vi "TimingLoop.vi"(8 "Error In":errorcluster, 11 "Message Queues":T1) -> (0 "Error Out":errorcluster)   [LabVIEW 2017, in "Server.lvlib" / "Timing.lvlib"]
doc: "This Loop is responsible for sending cyclic messages to MHL."
uses:
  Timing.lvlib
  Message Queue/CommReferences.ctl
  Message Queue/MessageCluster.ctl
  MessageSetList.ctl
  MessageSet.ctl
  <vilib>/Utility/error.llb/Error Cluster From Error Code.vi
  Message Queue/EnqueueMessage(Single).vi
  <vilib>/ErrorRing/Error Ring.xnode
  Message Queue/Message Queue.lvlib
  ErrorLogger/ErrorLogger.lvlib
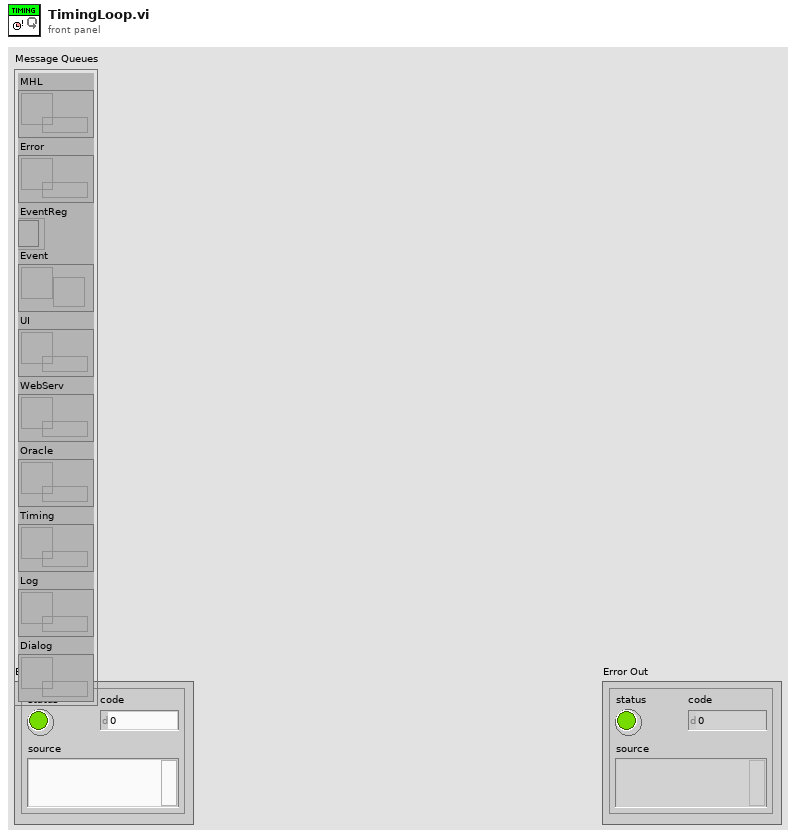
[diagram p1: front panel]
types:
  T1 = typedef "Server.lvlib/Message Queue.lvlib/CommReferences.ctl" = cluster{"MHL":refnum<queue>, "Error":refnum<queue>, "EventReg":refnum<event-registration>, "Event":refnum<user-event>, "UI":refnum<queue>, "WebServ":refnum<queue>, "Oracle":refnum<queue>, "Timing":refnum<queue>, "Log":refnum<queue>, "Dialog":refnum<queue>}
  T2 = typedef "Server.lvlib/Timing.lvlib/MessageSetList.ctl" = T3[]
  T3 = typedef "Server.lvlib/Timing.lvlib/MessageSet.ctl" = cluster{"MessageName":string, "Frequency (s)":dbl, "LastTime":timestamp}
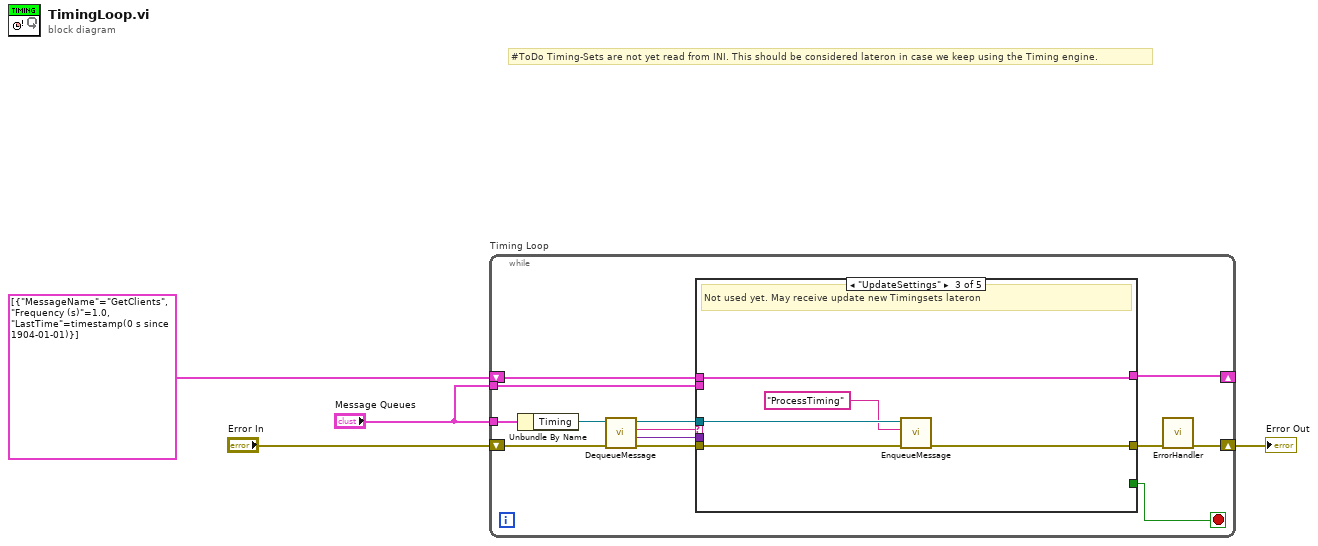
[diagram p0: block diagram]
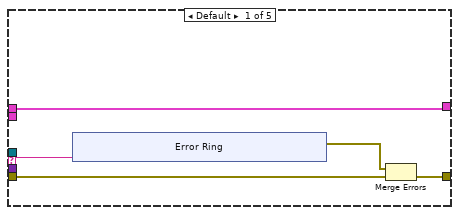
[diagram p2: hidden frame]
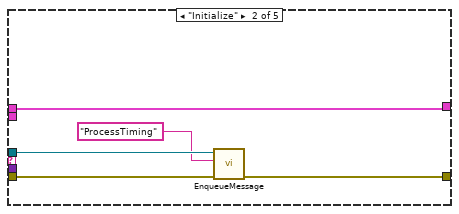
[diagram p3: hidden frame]
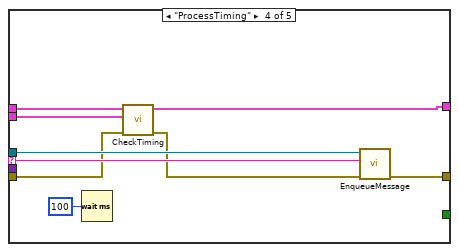
[diagram p4: hidden frame]
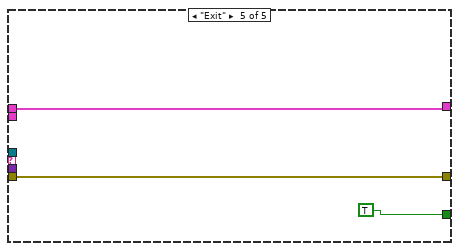
[diagram p5: hidden frame]
diagram:
  # "#ToDo Timing-Sets are not yet read from INI. This should be considered lateron in case we keep using the Timing engine."
  n1 = while "Timing Loop" {
    shift-right: [w6] -> w3
    shift-left: "Error In" -> [w17]
    tunnel: "Message Queues" -> [w12]
    shift-right: [w13] -> _
    shift-left: T2 [{"MessageName"="GetClients", "Frequency (s)"=1.0, "LastTime"=timestamp(0 s since 1904-01-01)}] -> [w14]
    tunnel: "Message Queues" -> [w5]
    stop <- w7 stop-if-true
    n2 = Unbundle By Name(w12) -> ("Timing"=w11:refnum<queue>)
    n3 = call "DequeueMessage.vi"("error in (no error)"=w17, "Message Queue"=w11) -> ("error out"=w15:errorcluster, "Message Data"=w9:variant, "Message"=w10:string, "dup Message Queue"=w8:refnum<queue>)  [unwired: 5 in, 1 out]
    n4 = case shown="\"UpdateSettings\"" w10 {
      selector: w10 -> [w20 _ _ w46 _]
      tunnel: [w19 w32 w37 w48 w51] -> w16
      tunnel: w15 -> [w22 w34 w39 w42 w51]
      tunnel: [w21 w33 w38 w44 w50] -> w13
      tunnel: w14 -> [w21 w33 w38 w45 w50]
      tunnel: w9 -> [_ _ _ _ _]
      tunnel: w8 -> [_ w31 w36 w47 _]
      tunnel: [_ _ _ _ TRUE] -> w7
      tunnel: w5 -> [_ _ _ w41 _]
      frame Default {
        n5 = xnode "Error Ring"("parameter 0"=w20) -> ("error out"=w18:errorcluster)
        n6 = Merge Errors(w18, w22) -> (w19:errorcluster)
      }
      frame "Initialize" {
        n7 = call-poly "EnqueueMessage.vi"("error in (no error)"=w34, "Message"="ProcessTiming", "Message Queue"=w31) -> ("error out"=w32:errorcluster)  [unwired: 7 in, 1 out]
      }
      frame "UpdateSettings" {
        # "Not used yet. May receive update new Timingsets lateron"
        n8 = call-poly "EnqueueMessage.vi"("error in (no error)"=w39, "Message"="ProcessTiming", "Message Queue"=w36) -> ("error out"=w37:errorcluster)  [unwired: 7 in, 1 out]
      }
      frame "ProcessTiming" {
        n9 = Wait (ms)(milliseconds to wait=u32 100) -> ()  [unwired: 1 out]
        n10 = call "CheckTiming.vi"("error in (no error)"=w42, "Message Queues"=w41, "MessageSetList"=w45) -> ("error out"=w40:errorcluster, "Array"=w44:T3[])  [unwired: 7 in]
        n11 = call-poly "EnqueueMessage.vi"("error in (no error)"=w40, "Message"=w46, "Message Queue"=w47) -> ("error out"=w48:errorcluster)  [unwired: 7 in, 1 out]
      }
      frame "Exit" {
      }
    }
    n12 = call "ErrorHandler.vi"("error in (no error)"=w16) -> ("error out"=w6:errorcluster)  [unwired: 10 in]
  }
  "Error Out" <- w3
